vi "test Set Even Parity by Index.vi"(8 "error in (no error)":errorcluster, 11 "TestCase in":refnum<class "Parity.lvclass">) -> (0 "error out":errorcluster, 3 "TestCase out":refnum<class "Parity.lvclass">)   [LabVIEW 2027, in "Parity.lvclass"]
uses:
  Parity.lvclass
  Source/Parity.ctl
  b79821fd-afdc-4fd3-a910-5010e2989e8e.vi
  C:/Program Files/National Instruments/LabVIEW 2027/vi.lib/addons/_JKI Toolkits/VI Tester/TestCase.llb/TestCase.lvclass
  <vilib>/addons/_JKI Toolkits/VI Tester/TestCase.llb/TestCase.lvclass
  Source/Encoding and Decoding.lvlib
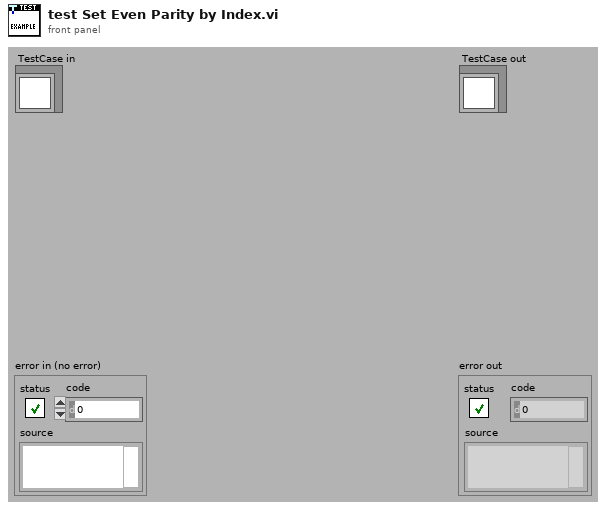
[diagram p1: front panel]
types:
  T1 = typedef "Encoding and Decoding.lvlib/Parity.ctl" = enum16{"Even", "Odd"}
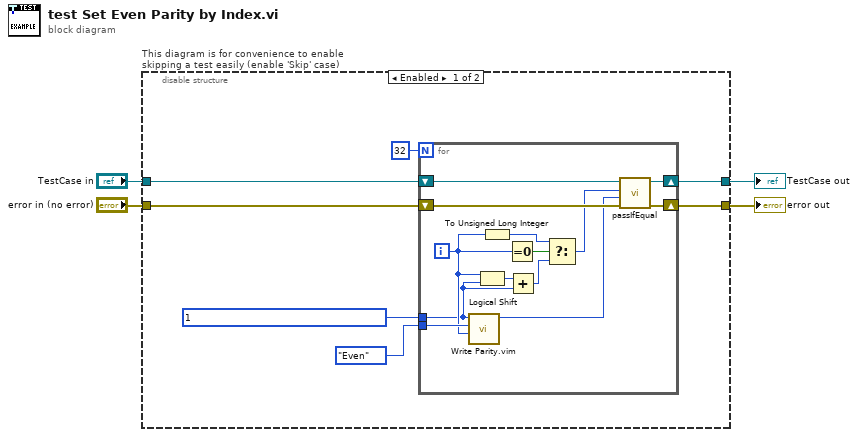
[diagram p0: block diagram]
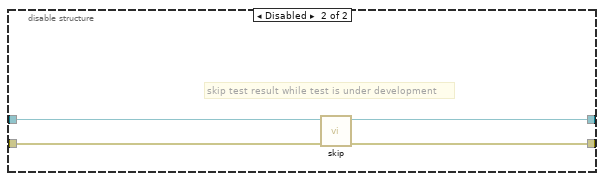
[diagram p2: hidden frame]
diagram:
  n1 = disable-structure "This diagram is for convenience to enable skipping a test easily (enable 'Skip' case)" shown="Enabled" {
    disable-tunnel: "TestCase in" -> [w11 w28]
    disable-tunnel: [w5 w26] -> w1
    disable-tunnel: [w6 w27] -> w3
    disable-tunnel: "error in (no error)" -> [w10 w25]
    frame Enabled {
      n2 = for {
        N: 32 -> [_]
        tunnel: u32 1 ("word in") -> [w12]
        tunnel: Parity."Even" ("parity") -> [w21]
        shift-right: [w20] -> w5
        shift-left: w11 -> [w24]
        shift-right: [w19] -> w6
        shift-left: w10 -> [w23]
        i -> [w16]
        n3 = call "Write Parity.vim"("parity index"=w16, "parity"=w21, "word in"=w12) -> ("word out"=w22:u32)  [unwired: 8 in]
        n4 = Logical Shift(y=w16, x=w12) -> (x << y=w18:u32)
        n5 = To Unsigned Long Integer(number=w16) -> (unsigned 32bit integer=w13:u32)
        n6 = Equal To 0?(x=w16) -> (x = 0?=w17:bool)
        n7 = Add(x=w18, y=w12) -> (x+y=w15:u32)
        n8 = Select(t=w13, s=w17, f=w15) -> (s? t:f=w14:u32)
        n9 = call-dynamic "passIfEqual.vi"("error in (no error)"=w23, "y"=w22, "x"=w14, "TestCase in"=w24) -> ("error out"=w19:errorcluster, "TestCase out"=w20:refnum<class "Parity.lvclass">)  [unwired: 6 in]
      }
    }
    frame Disabled {
      # "skip test result while test is under development"
      n10 = call <vilib>:"skip.vi"("error in (no error)"=w25, "TestCase in"=w28) -> ("error out"=w27:errorcluster, "TestCase out"=w26:refnum<class "Parity.lvclass">)  [unwired: 8 in]
    }
  }
  "error out" <- w3
  "TestCase out" <- w1
